vi "Sweep Sinewave Example 1.vi"(8 "Error In":errorcluster) -> (0 "Error Out":errorcluster)   [LabVIEW 2014]
uses:
  LabVIEW-Universal-Transcriptor-AD9850/AD9850.lvclass
panel:
  in  "w_clk":i32=8
  in  "fq_ud":i32=9
  in  "data":i32=10
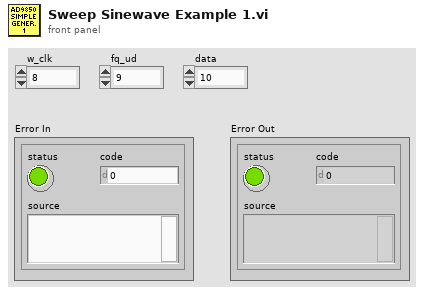
[diagram p1: front panel]
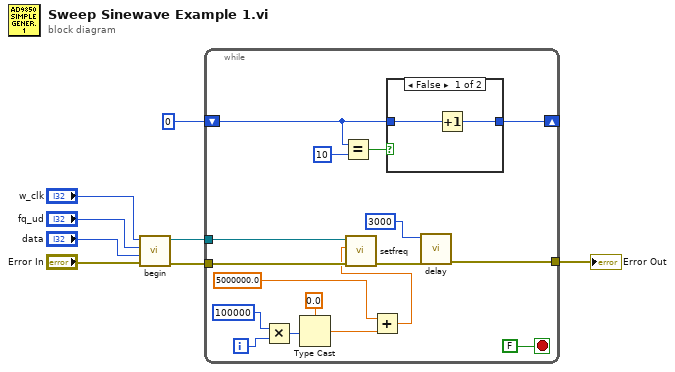
[diagram p0: block diagram]
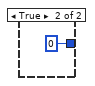
[diagram p2: hidden frame]
diagram:
  n1 = call "begin.vi"("error in (no error)"="Error In", "data"="data", "fq_ud"="fq_ud", "w_clk"="w_clk") -> ("error out"=w6:errorcluster, "AD9850 out"=w5:refnum<class "AD9850.lvclass">)  [unwired: 6 in]
  n2 = while {
    shift-right: [w22] -> _
    shift-left: 0 -> [w24]
    tunnel: w6 -> [w19]
    tunnel: w5 -> [w18]
    tunnel: [w13] -> w4
    i -> [w21]
    stop <- FALSE stop-if-true
    n3 = Multiply(x=100000, y=w21) -> (x*y=w17:i32)
    n4 = Type Cast(type=0.0, x=w17) -> (*(type *) &x=w12:dbl)
    n5 = Equal?(x=w24, y=10) -> (x = y?=w25:bool)
    n6 = Add(x=5000000.0, y=w12) -> (x+y=w9:dbl)
    n7 = call-dynamic "setfreq.vi"("error in (no error)"=w19, "frequency"=w9, "AD9850 in"=w18) -> ("error out"=w15:errorcluster)  [unwired: 7 in, 1 out]
    n8 = case shown="False" w25 {
      tunnel: w24 -> [w27 _]
      tunnel: [w26 0] -> w22
      frame False {
        n9 = Increment(x=w27) -> (x+1=w26:i32)
      }
      frame True {
      }
    }
    n10 = call <vilib>:"delay.vi"("Error In"=w15, "time (ms)"=3000) -> ("Error Out"=w13:errorcluster)  [unwired: 9 in]
  }
  "Error Out" <- w4
